vi "ABF_Read.vi"(4 "error in (no error)":errorcluster, 7 "Path of ABF file":path=path "D:/bme/abffile/demo3.abf") -> (0 "error out":errorcluster, 2 "File Paramters":T2, 3 "Whole Trace":sgl[][](graph))   [LabVIEW 2017]
panel:
  out "channel number":i32
  out "Header":T1
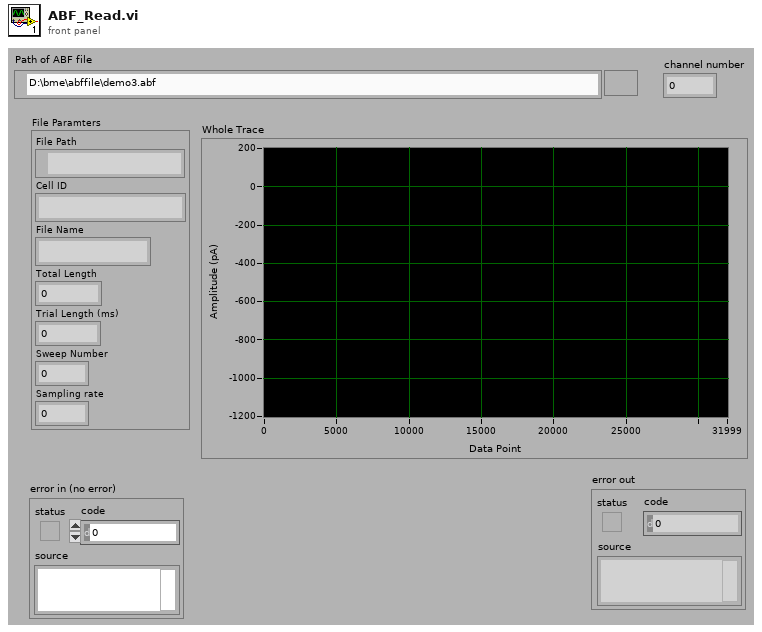
[diagram p1: front panel]
types:
  T1 = cluster{"AbfFormat":string, "fFileVersionNumber":sgl, "nOperationMode":i8, "IActualAcqLength":u32, "fNumPointsIgnored":i8, "IActualEpisodes":i32, "fADCSampleInterval":sgl, "INumSamplesPerEpisode":u32, "IEpisodesPerRun":u32, "fADCRange":sgl, "IADCResolution":u32}
  T2 = cluster{"File Path":path, "Cell ID":string, "File Name":string, "Total Length":i32, "Trial Length (ms)":dbl, "Sweep Number":dbl, "Sampling rate":dbl}
  T3 = enum16{"big-endian, network order", "native, host order", "little-endian"}
  T4 = cluster{"NumSamplePerEpisode":dbl, "sweepCount":u32, "dataRate":i32}
  T5 = cluster{"stripped path":path, "name":string, "name":string, dbl, "NumSamplePerEpisode":dbl, "sweepCount":u32, "dataRate":i32}
  T6 = cluster{"stripped path":path, "name":string, "name":string, dbl, dbl, dbl, "sampling rate":dbl}
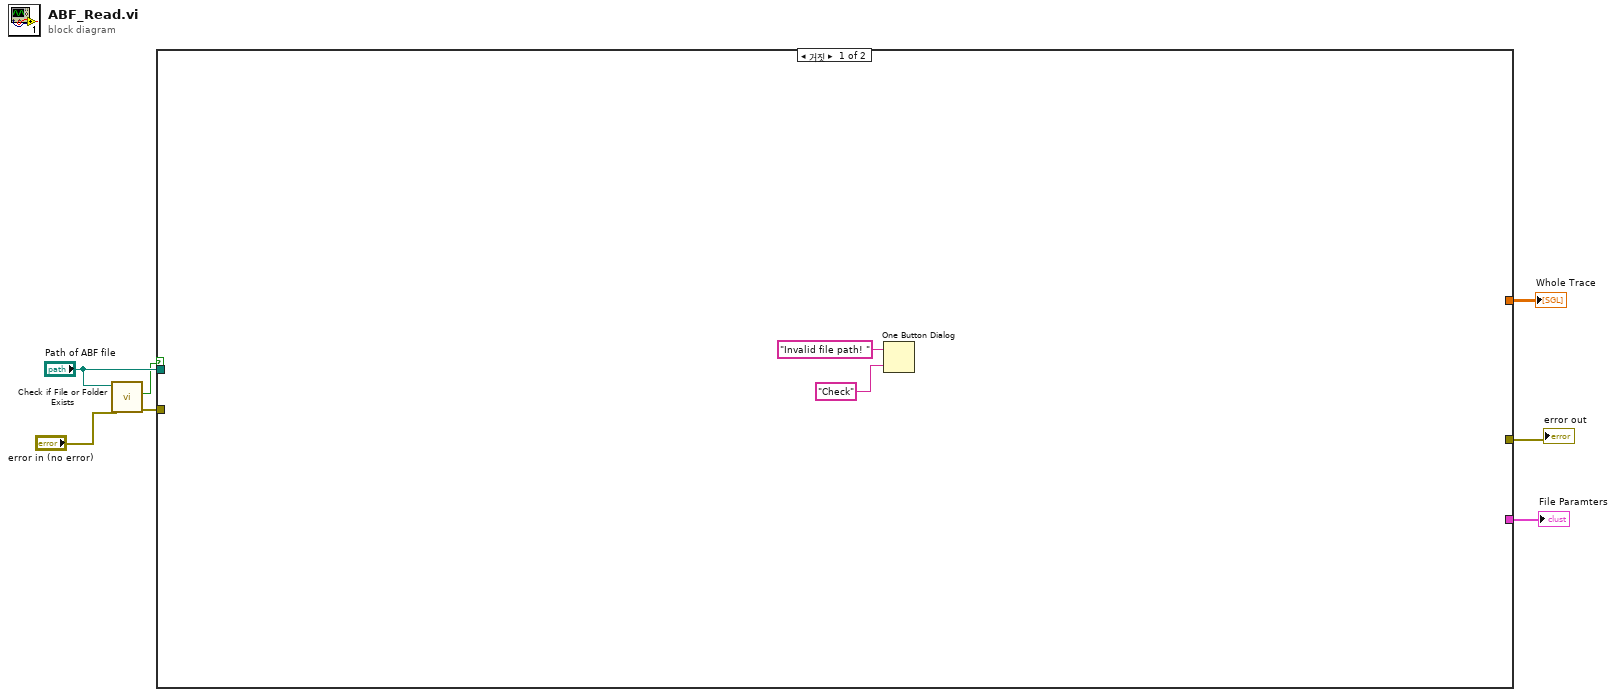
[diagram p0: block diagram]
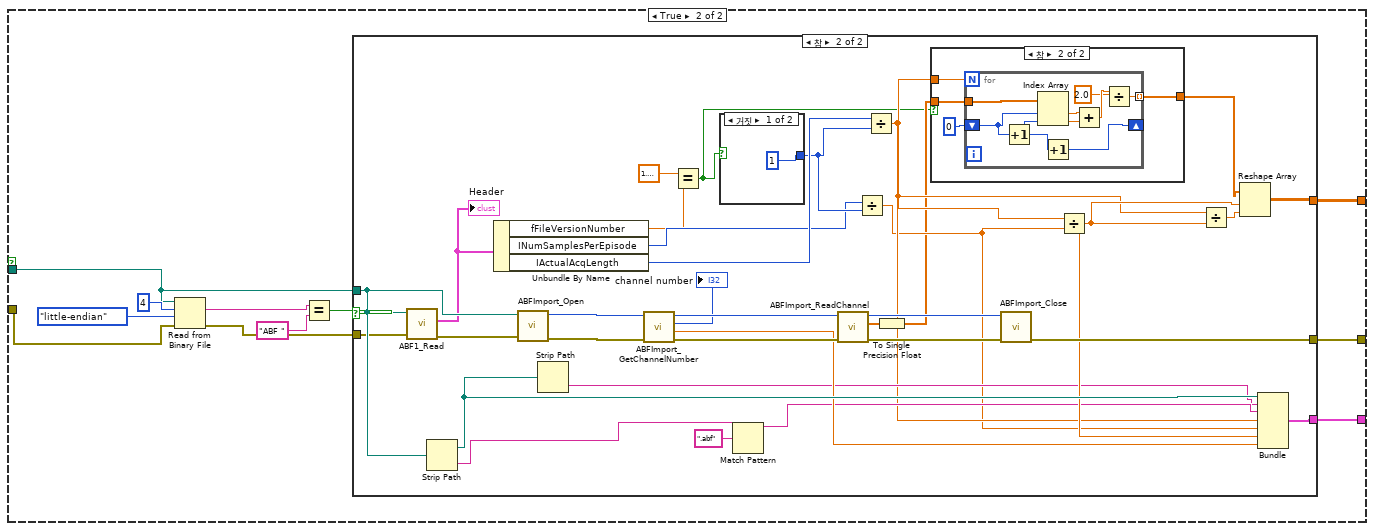
[diagram p2: hidden frame]
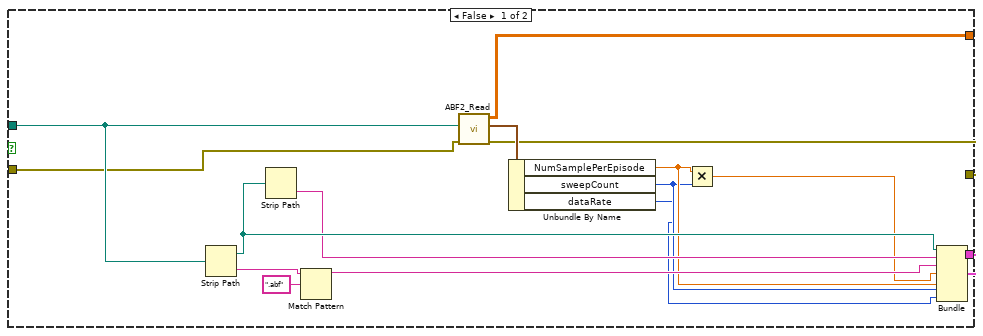
[diagram p3: hidden frame]
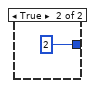
[diagram p5: hidden frame]
diagram:
  n1 = call <vilib>:"Check if File or Folder Exists.vi"("error in (no error)"="error in (no error)", "path"="Path of ABF file") -> ("error out"=w2:errorcluster, "file or folder exists?"=w1:bool)  [unwired: 7 in, 1 out]
  n2 = case shown="거짓" w1 {
    tunnel: [_ w20] -> w7
    tunnel: [_ w19] -> w6
    tunnel: [_ w12] -> w5
    tunnel: "Path of ABF file" -> [_ w11]
    tunnel: w2 -> [_ w10]
    frame False {
      n3 = One Button Dialog(message="Invalid file path! " ("메시지"), button name ("OK")="Check" ("버튼 이름(\"확인\")")) -> ()  [unwired: 1 out]
    }
    frame True {
      n4 = Read from Binary File(8:w10, 9:T3."little-endian" ("바이트 순서(0:big-endian, network order)"), 10:4 ("카운트(1)"), 11:w11) -> (0:w17:errorcluster, 2:w14:string)  [unwired: 2 in, 2 out]
      n5 = Equal?(x=w14, y="ABF ") -> (x = y?=w13:bool)
      n6 = case shown="참" w13 {
        tunnel: [w28 w63] -> w12
        tunnel: w11 -> [w34 w51]
        tunnel: [w32 w59] -> w20
        tunnel: w17 -> [w22 w50]
        tunnel: [w21 w57] -> w19
        frame False {
          n7 = Strip Path(path=w34) -> (stripped path=w31:path, name=w33:string)
          n8 = Strip Path(path=w31) -> (name=w30:string)  [unwired: 1 out]
          n9 = Match Pattern(string=w33, regular expression=".abf" ("정규식")) -> (before substring=w29:string)  [unwired: 1 in, 3 out]
          n10 = call "ABF2_Read.vi"("Error IN"=w22, "FilePath"=w34) -> ("Error OUT"=w21:errorcluster, "DataProperties"=w27:T4, "DataArray"=w28:sgl[][])  [unwired: 3 in]
          n11 = Unbundle By Name(w27) -> ("NumSamplePerEpisode"=w25:dbl, "sweepCount"=w24:u32, "dataRate"=w23:i32)
          n12 = Multiply(x=w25, y=w24) -> (x*y=w26:dbl)
          n13 = Bundle("stripped path"=w31, "name"=w30, "name"=w29, w26, "NumSamplePerEpisode"=w25, "sweepCount"=w24, "dataRate"=w23) -> (w32:T5)  [unwired: 1 in]
        }
        frame True {
          n14 = call "ABF1_Read.vi"("에러 입력"=w50, "FilePath"=w51) -> ("error out"=w49:errorcluster, "Header"=w48:T1)  [unwired: 4 in]
          "Header" <- w48
          n15 = Strip Path(path=w51) -> (stripped path=w60:path, name=w58:string)
          n16 = Unbundle By Name(w48) -> ("fFileVersionNumber"=w40:sgl, "INumSamplesPerEpisode"=w42:u32, "IActualAcqLength"=w45:u32)
          n17 = call "ABFImport_Open.vi"("error in (no error)"=w49, "abf file path"=w51) -> ("error out"=w66:errorcluster, "reference number"=w67:i32)  [unwired: 8 in]
          n18 = Strip Path(path=w60) -> (name=w53:string)  [unwired: 1 out]
          n19 = call "ABFImport_GetChannelNumber.vi"("error in (no error)"=w66, "reference number"=w67) -> ("error out"=w64:errorcluster, "sampling rate"=w56:dbl, "channel number"=→"channel number":i32, "reference out"=w65:i32)  [unwired: 6 in]
          n20 = Equal?(x=sgl 1.3, y=w40) -> (x = y?=w36:bool)
          n21 = case shown="거짓" w36 {
            tunnel: [u32 1 ("y") u32 2 ("y")] -> w43
            frame False {
            }
            frame True {
            }
          }
          n22 = Match Pattern(string=w58, regular expression=".abf" ("정규식")) -> (before substring=w54:string)  [unwired: 1 in, 3 out]
          n23 = call "ABFImport_ReadChannel.vi"("error in (no error)"=w64, "reference number"=w65) -> ("error out"=w68:errorcluster, "signal"=w46:sgl[], "reference out"=w61:i32)  [unwired: 7 in]
          n24 = Divide(x=w42, y=w43) -> (x/y=w41:dbl)
          n25 = Divide(x=w45, y=w43) -> (x/y=w44:dbl)
          n26 = To Single Precision Float(number=w46) -> (single precision float=w38:sgl[])
          n27 = case shown="참" w36 {
            tunnel: w44 -> [_ w72]
            tunnel: w38 -> [w69 w71]
            tunnel: [w69 w70] -> w37
            frame False {
            }
            frame True {
              n28 = for {
                N: w72 -> [_]
                tunnel: w71 -> [w82]
                shift-right: [w79] -> _
                shift-left: u32 0 ("y") -> [w81]
                tunnel: [w74] -> w70 mode=indexing
                n29 = Increment(x=w81) -> (x+1=w80:u32)
                n30 = Index Array(array=w82, index #1=w81, index #2=w80) -> (element #1=w78:sgl, element #2=w77:sgl)
                n31 = Increment(x=w80) -> (x+1=w79:u32)
                n32 = Add(x=w78, y=w77) -> (x+y=w76:sgl)
                n33 = Divide(x=w76, y=sgl 2.0) -> (x/y=w74:sgl)
              }
            }
          }
          n34 = call "ABFImport_Close.vi"("error in (no error)"=w68, "reference number"=w61) -> ("error out"=w57:errorcluster)  [unwired: 9 in]
          n35 = Divide(x=w44, y=w41) -> (x/y=w55:dbl)
          n36 = Divide(x=w44, y=w55) -> (x/y=w62:dbl)
          n37 = Reshape Array(w37, w55, w62) -> (w63:sgl[][])
          n38 = Bundle("stripped path"=w60, "name"=w53, "name"=w54, w44, w41, w55, "sampling rate"=w56) -> (w59:T6)  [unwired: 1 in]
        }
      }
    }
  }
  "Whole Trace" <- w5
  "File Paramters" <- w7
  "error out" <- w6
